vi "SplineHelp_GetCubicSpline_Calc3.vi"(4 "y-final-1":dbl, 6 "x-final-1":dbl, 8 "newWayPoints":T1[](array[typedef]) {"Y" format="%14.3f"; "X" format="%14.3f"}, 9 "dy-in":dbl[](array[numeric]), 11 "dx-in":dbl[](array[numeric])) -> (1 "dy-out":dbl[](array[numeric]), 3 "dx-out":dbl[](array[numeric]))   [LabVIEW 2019, in "Trajectory_Library.lvlib"]
doc: "Internal routine called by: SplineHelp_getCubicSplinesFromControlVectors.vi"
uses:
  Trajectory_Library.lvlib
  TypeDef/TRANSLATION2D.ctl
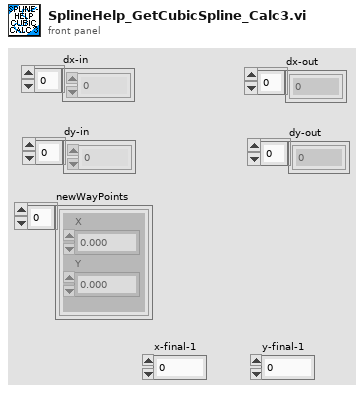
[diagram p1: front panel]
types:
  T1 = typedef "Trajectory_Library.lvlib/TRANSLATION2D.ctl" = cluster{"X":dbl, "Y":dbl}
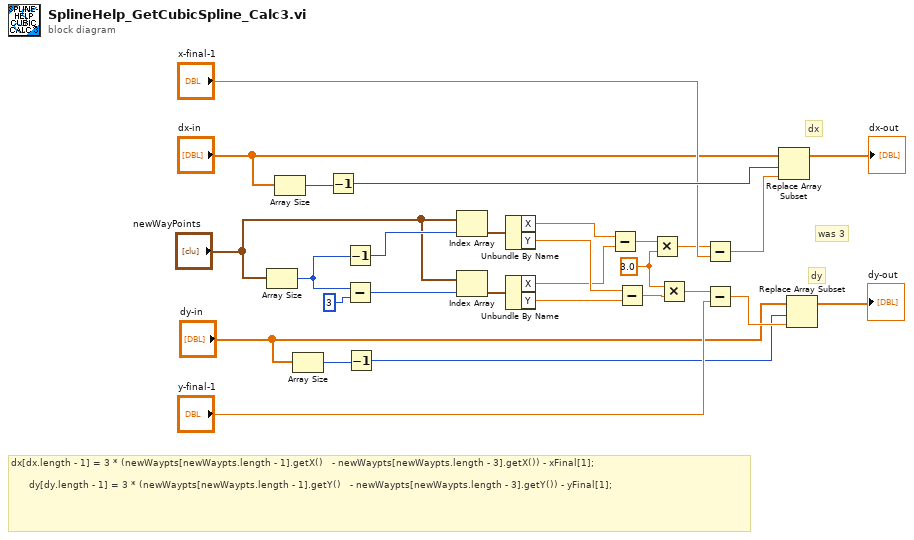
[diagram p0: block diagram]
diagram:
  w18 = 3.0
  # "was 3"
  # "dx[dx.length - 1] = 3 * (newWaypts[newWaypts.length - 1].getX()   - newWaypts[newWaypts.length - 3].getX()) - xFinal[1];\n\n      dy[dy.length - 1] = 3 * (newWaypts[newWaypts.length - 1].getY()   - newWaypts[newWaypts.length - 3].getY()) - yFinal[1];"
  # "dy"
  # "dx"
  n1 = Array Size(array="newWayPoints") -> (size(s)=w4:i32)
  n2 = Array Size(array="dx-in") -> (size(s)=w8:i32)
  n3 = Array Size(array="dy-in") -> (size(s)=w7:i32)
  n4 = Decrement(x=w8) -> (x-1=w28:i32)
  n5 = Decrement(x=w4) -> (x-1=w5:i32)
  n6 = Subtract(x=w4, y=3) -> (x-y=w1:i32)
  n7 = Decrement(x=w7) -> (x-1=w6:i32)
  n8 = Index Array(array="newWayPoints", index=w5) -> (element=w11:T1)
  n9 = Index Array(array="newWayPoints", index=w1) -> (element=w3:T1)
  n10 = Unbundle By Name(w11) -> ("X"=w12:dbl, "Y"=w14:dbl)
  n11 = Unbundle By Name(w3) -> ("X"=w13:dbl, "Y"=w15:dbl)
  n12 = Subtract(x=w12, y=w13) -> (x-y=w16:dbl)
  n13 = Subtract(x=w14, y=w15) -> (x-y=w17:dbl)
  n14 = Multiply(x=w16, y=w18) -> (x*y=w19:dbl)
  n15 = Multiply(x=w18, y=w17) -> (x*y=w20:dbl)
  n16 = Subtract(x=w19, y="x-final-1") -> (x-y=w27:dbl)
  n17 = Subtract(x=w20, y="y-final-1") -> (x-y=w26:dbl)
  n18 = Replace Array Subset(array="dx-in", new element=w27, index=w28) -> (→"dx-out":dbl[])
  n19 = Replace Array Subset(array="dy-in", new element=w26, index=w6) -> (→"dy-out":dbl[])
